vi "_DeviceAttributesInfo.vi"(0 "device name":string) -> (1 "error_stack":string[](array[string]), 2 "attributes_info":T1(array[cluster]), 3 "success":bool)   [LabVIEW 2014, in "tango.lvlib"]
uses:
  tango.lvlib
  tango_binding.so
panel:
  out "error_stack (internal)":string[](array[string])
  out "success (internal)":bool
  # "AttributeInfo.r/w access\n-----------------------\n\tREAD = 0\n READ_WITH_WRITE = 1\n WRITE = 2\n READ_WRITE = 3"
  # "AttributeInfo.data-type\n-----------------------\n\tDEV_VOID = 0\n\tDEV_BOOLEAN = 1\n\tDEV_SHORT = 2\n\tDEV_LONG = 3\n\tDEV_FLOAT = 4\n\tDEV_DOUBLE = 5\n\tDEV_USHORT = 6\n\tDEV_ULONG = 7\n\tDEV_STRING = 8\n\tDEVVAR_CHARARRAY = 9\n\tDEVVAR_SHORTARRAY = 10\n\tDEVVAR_LONGARRAY = 11\n\tDEVVAR_FLOATARRAY = 12\n\tDEVVAR_DOUBLEARRAY = 13\n\tDEVVAR_USHORTARRAY = 14\n\tDEVVAR_ULONGARRAY = 15\n\tDEVVAR_STRINGARRAY = 16\n\tDEVVAR_LONGSTRINGARRAY = 17\n\tDEVVAR_DOUBLESTRINGARRAY = 18\n\tDEV_STATE = 19\n\tCONST_DEV_STRING = 20\n\tDEVVAR_BOOLEANARRAY = 21\n\tDEV_UCHAR = 22\n\tDEV_LONG64 = 23\n\tDEV_ULONG64 = 24\n\tDEVVAR_LONG64ARRAY = 25\n\tDEVVAR_ULONG64ARRAY = 26\n\tDEV_INT = 27\n\tDEV_ENCODED = 28"
  # "AttributeInfo.format\n-----------------------\n\tSCALAR = 0\n SPECTRUM = 1\n IMAGE = 2"
  # "AttributeInfo.level\n-----------------------\n\tOPERATOR = 0\n EXPERT = 1"
  # "This Vi is deprecated and only maintained for backward compatibility. Please use  _TangoAttributesInfo instead."
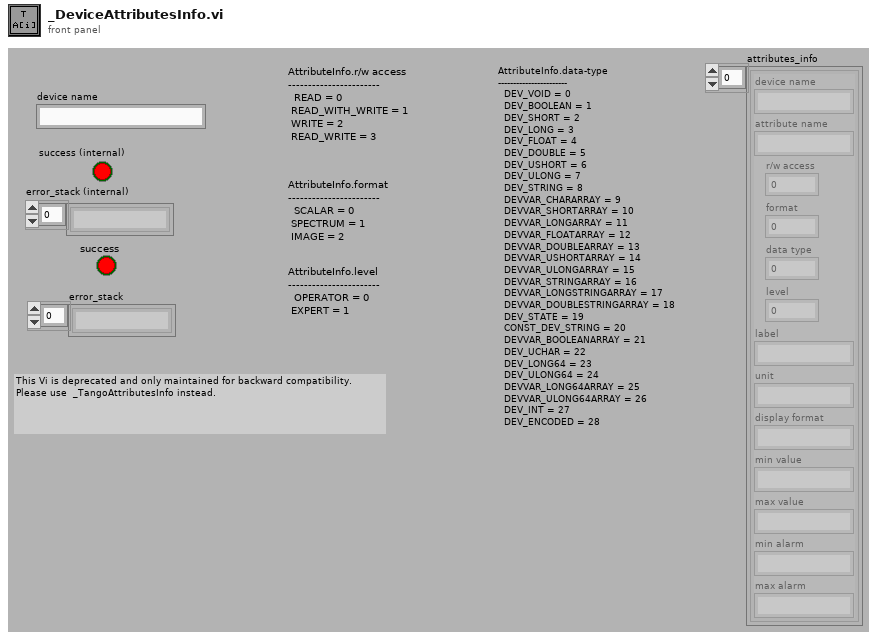
[diagram p1: front panel]
types:
  T1 = cluster{"device name":string, "attribute name":string, "r/w access":i16, "format":i16, "data type":i16, "level":i16, "label":string, "unit":string, "display format":string, "min value":string, "max value":string, "min alarm":string, "max alarm":string}[]
  T2 = typedef "tango.lvlib/_AttributeInfo_t.ctl" = cluster{"device name":string, "attribute name":string, "r/w access":T3, "format":T4, "data type":T5, "level":T6, "label":string, "unit":string, "display format":string, "min value":string, "max value":string, "min alarm":string, "max alarm":string}
  T3 = typedef "tango.lvlib/_AttributeAccess_t.ctl" = enum16{"READ", "READ_WITH_WRITE", "WRITE", "READ_WRITE", "UNKNOWN_ACCESS_TYPE"}
  T4 = typedef "tango.lvlib/_AttributeFormat_t.ctl" = enum16{"SCALAR", "SPECTRUM", "IMAGE", "UNKNOWN_FORMAT"}
  T5 = typedef "tango.lvlib/_TangoDataType_t.ctl" = enum16{"VOID", "BOOLEAN", "SHORT", "LONG", "FLOAT", "DOUBLE", "USHORT", "ULONG", "STRING", "CHAR_ARRAY", "SHORT_ARRAY", "LONG_ARRAY", "FLOAT_ARRAY", "DOUBLE_ARRAY", "USHORT_ARRAY", "ULONG_ARRAY", "STRING_ARRAY", "LONG_STRING_ARRAY", "DOUBLE_STRING_ARRAY", "STATE", "CONST_STRING", "BOOLEAN_ARRAY", "UCHAR", "LONG64", "ULONG64", "LONG64_ARRAY", "ULONG64_ARRAY", "INT (not supported)", "ENCODED (not supported)", "ENUM", "PIPE_BLOB (not supported)", "STATE_ARRAY", "UNKNOW_DATA_TYPE"}
  T6 = typedef "tango.lvlib/_AttributeLevel_t.ctl" = enum16{"OPERATOR", "EXPERT", "UNKNOWN_LEVEL"}
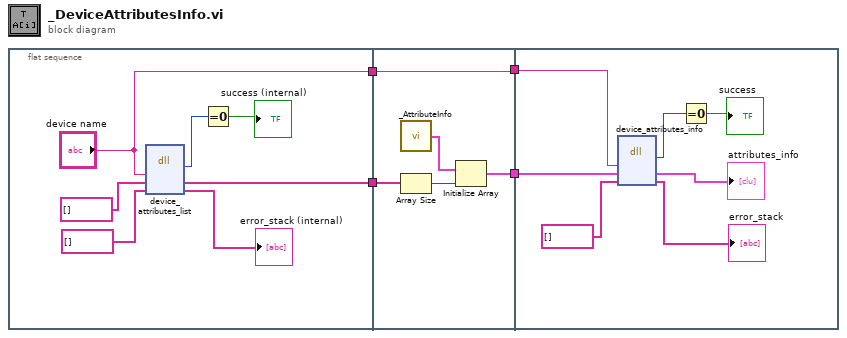
[diagram p0: block diagram]
diagram:
  n1 = flat-sequence {
    tunnel: [w7] -> w4
    tunnel: ["device name"] -> w1
    tunnel: w4 -> [w16]
    tunnel: [w13] -> w3
    tunnel: [w12] -> w2
    tunnel: w1 -> [w12]
    tunnel: w3 -> [w20]
    tunnel: w2 -> [w19]
    frame #0 {
      n2 = dll-call lib="tango_binding.*" fn="device_attributes_list"("dev_name"="device name", "attributes_list"=string[] [] ("Error Stack"), "error_stack"=string[] [] ("Error Stack")) -> ("return type"=w9:i32, "attributes_list"=w7:string[], "error_stack"=→"error_stack (internal)":string[])  [unwired: 4 in, 2 out]
      n3 = Equal To 0?(x=w9) -> (x = 0?=→"success (internal)":bool)
    }
    frame #1 {
      n4 = call "_AttributeInfo.vi"() -> ("attribute info"=w14:T2)  [unwired: 15 in]
      n5 = Array Size(array=w16) -> (size(s)=w15:i32)
      n6 = Initialize Array(w14, w15) -> (w13:T2[])
    }
    frame #2 {
      n7 = dll-call lib="tango_binding.*" fn="device_attributes_info"("dev_name"=w19, "attributes_info"=w20, "error_stack"=string[] [] ("Error Stack")) -> ("return type"=w21:i32, "attributes_info"=→"attributes_info":T2[], "error_stack"=→"error_stack":string[])  [unwired: 4 in, 2 out]
      n8 = Equal To 0?(x=w21) -> (x = 0?=→"success":bool)
    }
  }
